vi "PH_Get6PInformation.PC Get Info.vi"(2 "PCS Motion List Ref":refnum<vi>, 5 "error in":errorcluster) -> (19 "error out":errorcluster)   [LabVIEW 2014, in "PH_Get6PInformation.lvlib"]
doc: "This is the proc case \"get information\"."
uses:
  PH_Get6PInformation.lvlib
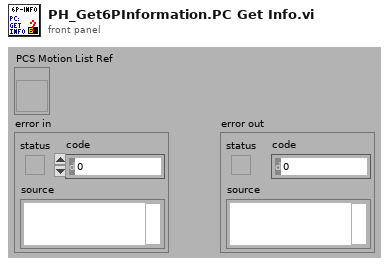
[diagram p1: front panel]
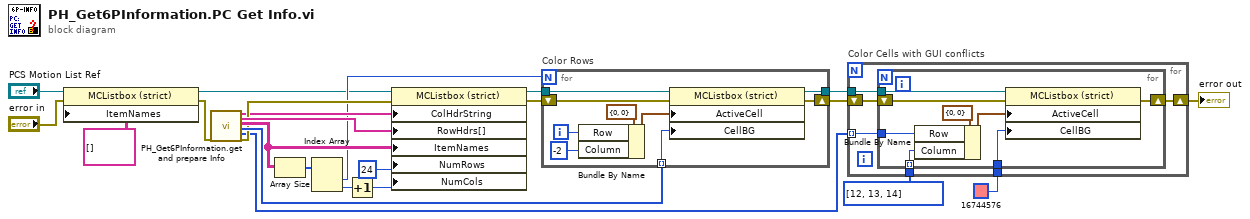
[diagram p0: block diagram]
diagram:
  n1 = property class="MCListbox (strict)"(reference="PCS Motion List Ref", error in="error in", "ItemNames"=string[][] [] ("Value")) -> (reference out=w1:refnum<vi>, error out=w15:errorcluster)
  n2 = call "PH_Get6PInformation.get and prepare Info.vi"("error in"=w15) -> ("ColHdrs[]"=w18:string[], "RowHdrs[]"=w21:string[], "ItemNames"=w22:string[][], "Row Cell BG"=w20:u32[], "Rows with GUI conflict"=w17:i32[], "error out"=w19:errorcluster)  [unwired: 13 in]
  n3 = Array Size(array=w22) -> (size(s)=w12:i32[])
  n4 = Index Array(array=w12) -> (element #1=w6:i32, element #2=w7:i32)  [unwired: 2 in]
  n5 = Increment(x=w7) -> (x+1=w10:i32)
  n6 = property class="MCListbox (strict)"(reference=w1, error in=w19, "ColHdrString"=w18, "RowHdrs[]"=w21, "ItemNames"=w22, "NumRows"=u32 24 ("Number of Rows"), "NumCols"=w10) -> (reference out=w8:refnum<vi>, error out=w9:errorcluster)
  n7 = for "Color Rows" {
    N: w6 -> [_]
    tunnel: w8 -> [w30]
    shift-right: [w31] -> w5
    shift-left: w9 -> [w32]
    tunnel: w20 -> [w27] mode=indexing
    tunnel: [w24] -> w4
    i -> [w26]
    n8 = Bundle By Name(cluster=cluster{"Row":i32, "Column":i32} {"Row"=0, "Column"=0} ("Active Cell:Active Cell"), "Row"=w26, "Column"=-2 ("Row")) -> (w29:cluster{"Row":i32, "Column":i32})
    n9 = property class="MCListbox (strict)"(reference=w30, error in=w32, "ActiveCell"=w29, "CellBG"=w27) -> (reference out=w24:refnum<vi>, error out=w31:errorcluster)
  }
  n10 = for "Color Cells with GUI conflicts" {
    tunnel: w4 -> [w36]
    tunnel: w17 -> [w35] mode=indexing
    shift-right: [w37] -> w23
    shift-left: w5 -> [w38]
    tunnel: i32[] [12, 13, 14] -> [w34]
    tunnel: u32 16744576 ("Color Box") -> [w33]
    n11 = for "Color Cells with GUI conflicts" {
      tunnel: w36 -> [w44]
      shift-right: [w45] -> w37
      shift-left: w38 -> [w46]
      tunnel: w33 -> [w41]
      tunnel: w35 -> [w40]
      tunnel: w34 -> [w39] mode=indexing
      n12 = Bundle By Name(cluster=cluster{"Row":i32, "Column":i32} {"Row"=0, "Column"=0} ("Active Cell:Active Cell"), "Row"=w40, "Column"=w39) -> (w43:cluster{"Row":i32, "Column":i32})
      n13 = property class="MCListbox (strict)"(reference=w44, error in=w46, "ActiveCell"=w43, "CellBG"=w41) -> (error out=w45:errorcluster)  [unwired: 1 out]
    }
  }
  "error out" <- w23
